vi "movavg.vi"(4 "Numeric in":i32, 6 "Length":i32, 9 "Array in":dbl[](array[numeric]), 10 "y":dbl, 11 "data":dbl) -> (2 "Array out":dbl[](array[numeric]), 3 "Numeric out":dbl)   [LabVIEW 2011]
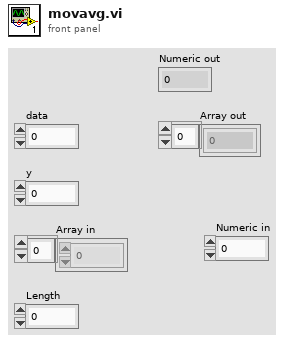
[diagram p1: front panel]
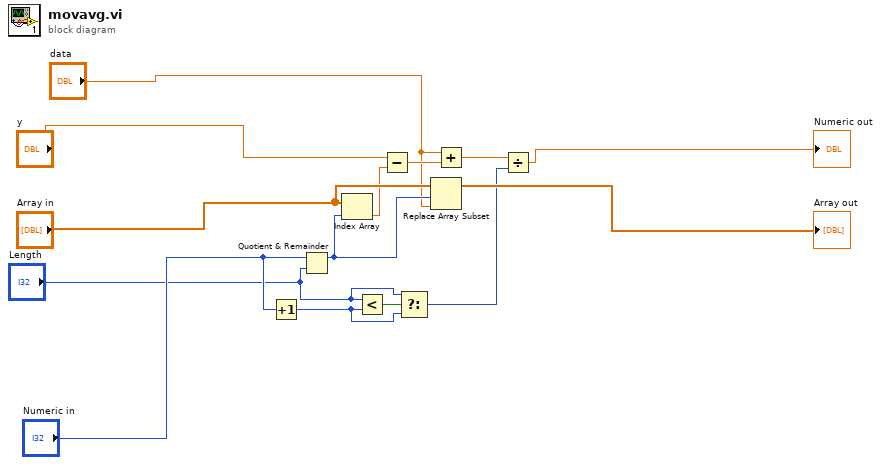
[diagram p0: block diagram]
diagram:
  n1 = Increment(x="Numeric in") -> (x+1=w7:i32)
  n2 = Quotient & Remainder(x="Numeric in", y="Length") -> (x-y*floor(x/y)=w4:i32)  [unwired: 1 out]
  n3 = Index Array(array="Array in", index=w4) -> (element=w2:dbl)
  n4 = Less?(x="Length", y=w7) -> (x < y?=w5:bool)
  n5 = Subtract(x="y", y=w2) -> (x-y=w3:dbl)
  n6 = Select(t="Length", s=w5, f=w7) -> (s? t:f=w6:i32)
  n7 = Replace Array Subset(array="Array in", new element="data", index=w4) -> (→"Array out":dbl[])
  n8 = Add(x="data", y=w3) -> (x+y=w13:dbl)
  n9 = Divide(x=w13, y=w6) -> (x/y=→"Numeric out":dbl)
